vi "Read module async property.vi"(7 "Module ID":string, 8 "error in":errorcluster, 11 "Standard Engine Repo Data in":refnum<class "Standard Engine Configuration.lvclass">) -> (0 "error out":errorcluster, 2 "async?":bool, 3 "Standard Engine Repo Data out":refnum<class "Standard Engine Configuration.lvclass">)   [LabVIEW 2013, in "Standard Engine Configuration.lvclass"]
doc: "Returns whether or not a specific module has been configured to run asynchronously by the engine."
uses:
  Standard Engine Configuration.lvclass
  Standard Engine Configuration.lvclass/Standard Engine Configuration.ctl
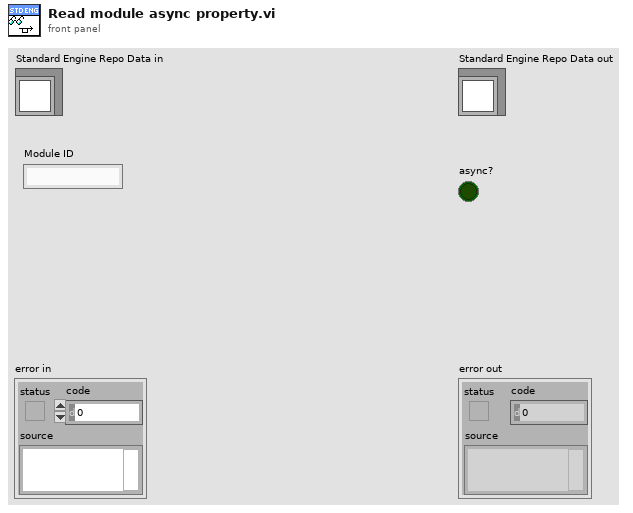
[diagram p1: front panel]
types:
  T1 = typedef "Standard Engine Configuration.lvclass/Module Specific Configuration.ctl" = cluster{"Module ID":string, "Module Decimation":T2, "error tag":string, "error responses":T3}
  T2 = typedef "Standard Engine Configuration.lvclass/Module Decimation.ctl" = cluster{"Decimation":u16, "Offset":u16, "sort order":i32, "async?":bool}
  T3 = typedef "Standard Engine Configuration.lvclass/error responses.ctl" = cluster{"unknown":T4, "trivial":T4, "critical":T4, "recoverable":T4}
  T4 = typedef "Standard Engine Configuration.lvclass/error options.ctl" = cluster{"clear":bool, "notify":bool, "remove module":bool, "abort engine":bool, "go to safe state":bool, "recover module":bool}
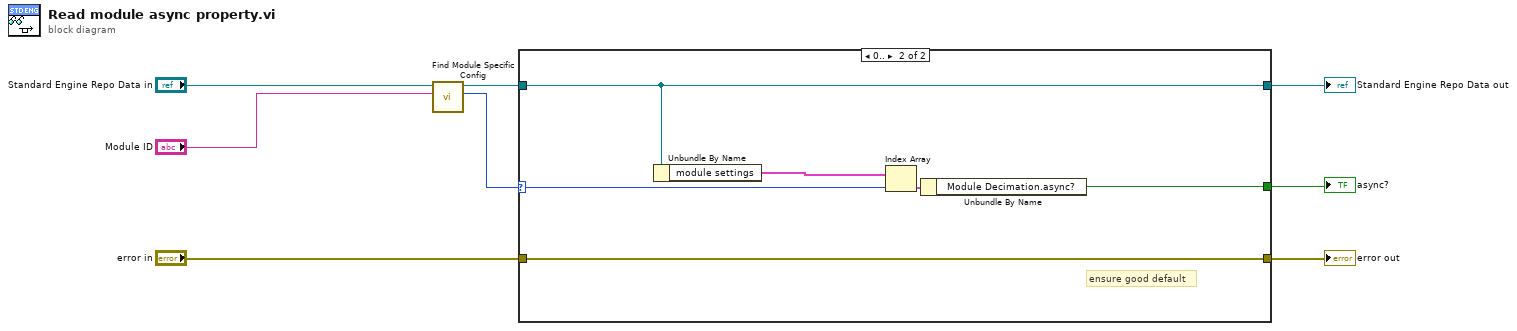
[diagram p0: block diagram]
diagram:
  n1 = call "Find Module Specific Config.vi"("Module ID"="Module ID", "Standard Engine Repo Data in"="Standard Engine Repo Data in") -> ("Index"=w1:i32, "Standard Engine Repo Data out"=w2:refnum<class "Standard Engine Configuration.lvclass">)  [unwired: 8 in]
  n2 = case shown="0.." w1 {
    selector: w1 -> [_ w13]
    tunnel: w2 -> [w10 w14]
    tunnel: "error in" -> [w9 w12]
    tunnel: [w9 w12] -> w4
    tunnel: [w10 w14] -> w6
    tunnel: [_ w11] -> w3
    frame ..-1 {
    }
    frame 0.. {
      # "ensure good default"
      n3 = Unbundle By Name(w14) -> ("module settings"=w16:T1[])
      n4 = Index Array(array=w16, index=w13) -> (element=w15:T1)
      n5 = Unbundle By Name(w15) -> ("Module Decimation.async?"=w11:bool)
    }
  }
  "error out" <- w4
  "Standard Engine Repo Data out" <- w6
  "async?" <- w3
